vi "U6 Single IO Example.vi"() -> (0 "error out":errorcluster)   [LabVIEW 2021]
panel:
  in  "IOType Ring":u16(ring)=3 items=["LJ_ioGET_AIN", "LJ_ioGET_AIN_DIFF", "LJ_ioPUT_DAC", "LJ_ioGET_DIGITAL_BIT", "LJ_ioGET_DIGITAL_PORT", "LJ_ioPUT_DIGITAL_BIT", "LJ_ioPUT_DIGITAL_PORT"]
  in  "x1":i32
  in  "FirstFound":bool=TRUE
  in  "Address":string="1"
  in  "Value Write":dbl format="%.3f"
  out "Error Message":string
  out "Value Read":dbl format="%.6f"
  in  "Channel #":i32
  # "Reads 1 input or writes 1 output.  Use \"U3 Pin Configuration Example.vi\" to set pins to digital\nor analog."
  # "Used for digital port IOtypes where\nx1 specifies the # of bits and then\nChannel # specifies starting channel.\nFor differential AIN, x1 specifies\nnegative channel."
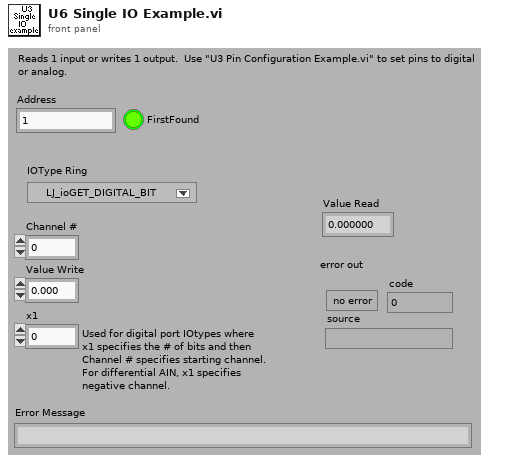
[diagram p1: front panel]
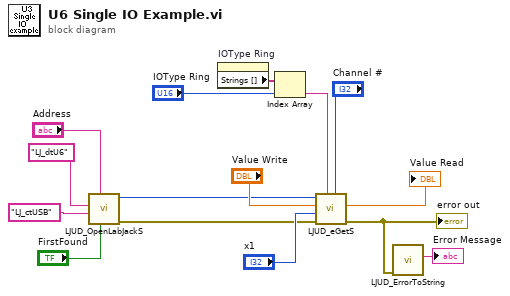
[diagram p0: block diagram]
diagram:
  n1 = call "LJUD_OpenLabJackS.vi"("FirstFound"="FirstFound", "Address"="Address", "ConnectionType"="LJ_ctUSB", "DeviceType"="LJ_dtU6") -> ("error out"=w1:errorcluster, "Handle"=w2:i32)  [unwired: 5 in, 1 out]
  n2 = property on="IOType Ring" class="Ring (strict)"() -> ("Strings []"=w7:string[])  [unwired: 2 in, 2 out]
  n3 = Index Array(array=w7, index="IOType Ring") -> (element=w5:string)
  n4 = call "LJUD_eGetS.vi"("Channel"="Channel #", "IOType"=w5, "error in"=w1, "x1"="x1", "Value Write"="Value Write", "Handle In"=w2) -> ("error out"=w12:errorcluster, "Value Read"=→"Value Read":dbl)  [unwired: 3 in, 1 out]
  "error out" <- w12
  n5 = call "LJUD_ErrorToString.vi"("error in"=w12) -> ("String"=→"Error Message":string)  [unwired: 10 in]
